vi "stations POST to INSTRUMENTS.vi"(5 "POST (empty)":T2) -> (2 "INSTRUMENTS on Station":T1[](array[typedef]))   [LabVIEW 2011]
uses:
  ITK EXT/utils/keyedarr.llb/Keyed Array.ctl
  server/database/Stations/Instruments/Instrument Record.ctl
  ITK EXT/utils/strutil.llb/Case Matching.ctl
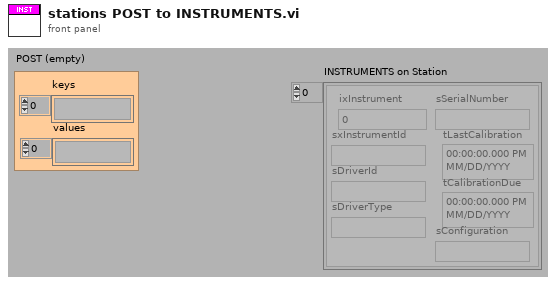
[diagram p1: front panel]
types:
  T1 = typedef "Instrument Record.ctl" = cluster{"ixInstrument":i32, "sxInstrumentId":string, "sDriverId":string, "sDriverType":string, "sSerialNumber":string, "tLastCalibration":timestamp, "tCalibrationDue":timestamp, "sConfiguration":string}
  T2 = typedef "Keyed Array.ctl" = cluster{"keys":string[], "values":string[]}
  T3 = typedef "Case Matching.ctl" = enum16{"a != A", "a == A", "system"}
  T4 = cluster{"[0]":string, "[1]":string, "[2]":string, "[3]":string, "[4]":string, "[5]":string, "[6]":string, "[7]":string}
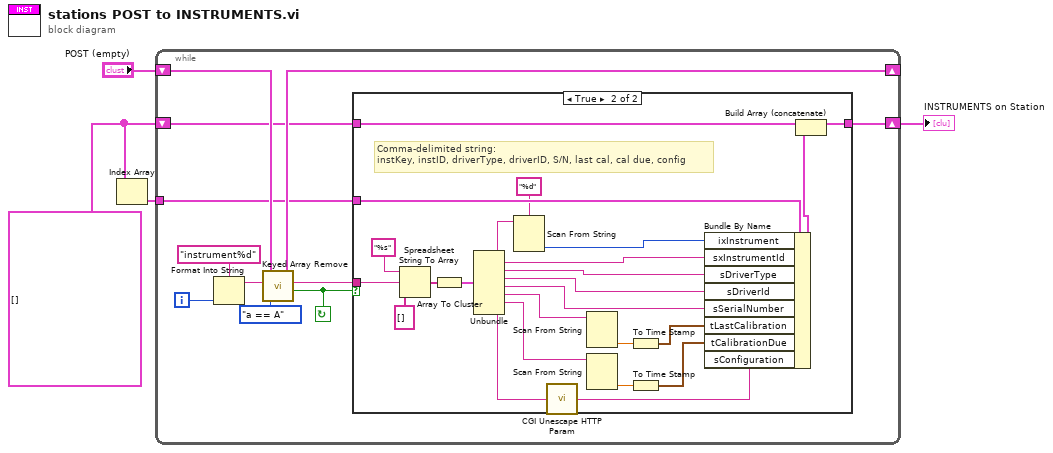
[diagram p0: block diagram]
diagram:
  w3 = T1[] []
  n1 = Index Array(array=w3) -> (element=w2:T1)  [unwired: 1 in]
  n2 = while {
    shift-right: [w10] -> _
    shift-left: "POST (empty)" -> [w15]
    shift-right: [w6] -> w1
    shift-left: w3 -> [w7]
    tunnel: w2 -> [w5]
    i -> [w11]
    stop <- w9 continue-if-true
    n3 = Format Into String(format string="instrument%d", w11) -> (resulting string=w12:string)  [unwired: 2 in, 1 out]
    n4 = call "Keyed Array Remove.vi"("case matching (sensitive)"=Case_Matching."a == A", "key"=w12, "array in"=w15) -> ("valid key"=w9:bool, "value"=w8:string, "array out"=w10:T2)  [unwired: 2 out]
    n5 = case shown="True" w9 {
      tunnel: w8 -> [_ w35]
      tunnel: w7 -> [w16 w40]
      tunnel: [w16 w39] -> w6
      tunnel: w5 -> [_ w38]
      frame False {
      }
      frame True {
        # "Comma-delimited string:\ninstKey, instID, driverType, driverID, S/N, last cal, cal due, config"
        n6 = Spreadsheet String To Array(format string="%s", spreadsheet string=w35, array type (2D Dbl)=string[] []) -> (array=w32:string[])  [unwired: 1 out]
        n7 = Array To Cluster(array=w32) -> (cluster=w31:T4)
        n8 = Unbundle(w31) -> ("[0]"=w30:string, "[1]"=w27:string, "[2]"=w26:string, "[3]"=w25:string, "[4]"=w24:string, "[5]"=w22:string, "[6]"=w17:string, "[7]"=w23:string)
        n9 = Scan From String(format string="%d", input string=w30) -> (output 1=w29:i32)  [unwired: 2 in, 4 out]
        n10 = call "CGI Unescape HTTP Param.vi"("url-encoded string"=w23) -> ("string"=w36:string)
        n11 = Scan From String(input string=w22) -> (output 1=w21:dbl)  [unwired: 3 in, 4 out]
        n12 = Scan From String(input string=w17) -> (output 1=w19:dbl)  [unwired: 3 in, 4 out]
        n13 = To Time Stamp(1:w21) -> (0:w20:timestamp)
        n14 = To Time Stamp(1:w19) -> (0:w18:timestamp)
        n15 = Bundle By Name(cluster=w38, "ixInstrument"=w29, "sxInstrumentId"=w27, "sDriverType"=w26, "sDriverId"=w25, "sSerialNumber"=w24, "tLastCalibration"=w20, "tCalibrationDue"=w18, "sConfiguration"=w36) -> (w37:T1)
        n16 = Build Array (concatenate)(w40, w37) -> (w39:T1[])
      }
    }
  }
  "INSTRUMENTS on Station" <- w1
